vi "Pockels-Initialise sequence for funct acq.vi"(9 "Cluster":T1={"Pockels ON \"Pre\" (samples)"=0, "Direction (+-Inf)"=enum."Toward +Inf", "Additional duration to stay ON (samples)"=0, "Not the last ROI"=FALSE}) -> (1 "Count towards trigger target (ms)":dbl format="%#_9g", 2 "Excess (us)":dbl format="%#_9g", 3 "waveform out":waveform(dbl)(graph))   [LabVIEW 2017]
uses:
  Typedefs/Pockels modulation Internal cluster 1.ctl
  Typedefs/Rounding type.ctl
  Typedefs/Imaging Protocols enum.ctl
  Global Variables/General Globals.vi
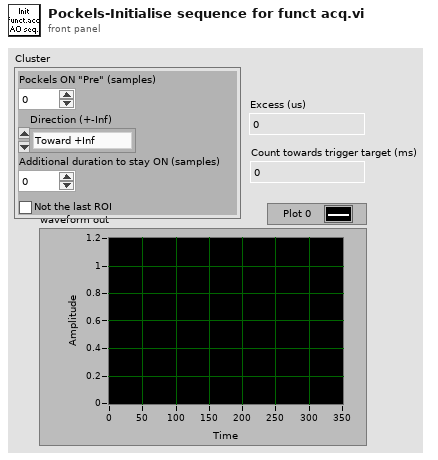
[diagram p1: front panel]
types:
  T1 = typedef "Pockels modulation Internal cluster 1.ctl" = cluster{"Pockels ON \"Pre\" (samples)":i32, "Direction (+-Inf)":T2, "Additional duration to stay ON (samples)":i32, "Not the last ROI":bool}
  T2 = typedef "Rounding type.ctl" = enum16{"No rounding", "Toward +Inf", "Toward -Inf"}
  T3 = typedef "Imaging Protocols enum.ctl" = enum16{"AOL Z-Stack", "Motor Z Stack", "Functional Acquisition", "Single Plane Acquisition", "Volume Acquisition", "Live Imaging", "Live Plane Imaging", "Live Volume Imaging"}
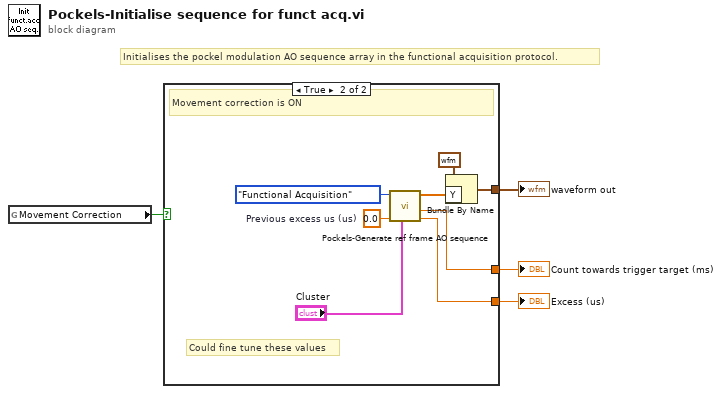
[diagram p0: block diagram]
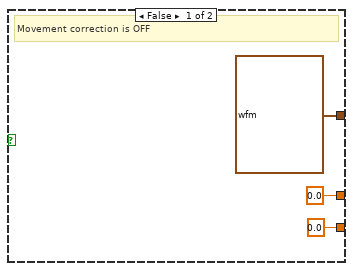
[diagram p2: hidden frame]
diagram:
  # "Initialises the pockel modulation AO sequence array in the functional acquisition protocol."
  n1 = global read "General Globals.vi" "Movement Correction"() -> (w3:bool)
  n2 = case shown="True" w3 {
    tunnel: [waveform(dbl) {"t0"=timestamp(0 s since 1904-01-01), "dt"=0.0, "Y"=[]} ("waveform out") w14] -> w4
    tunnel: [0.0 ("Count towards trigger target (us)") w11] -> w2
    tunnel: [0.0 ("Count towards trigger target (us)") w10] -> w1
    frame False {
      # "Movement correction is OFF"
    }
    frame True {
      w9 = 0.0  # Previous excess us (us)
      # "Could fine tune these values"
      # "Movement correction is ON"
      n3 = call "Pockels-Generate ref frame AO sequence.vi"("Cluster"="Cluster", "Previous excess us (us)"=w9, "Imaging Protocol"=Imaging_Protocols_enum."Functional Acquisition") -> ("Excess (us)"=w10:dbl, "Output sequence length (ms) (corrected for input excess)"=w11:dbl, "Pockels modulation sequence"=w15:dbl[])  [unwired: 4 in, 2 out]
      n4 = Bundle By Name ("Build Waveform")(cluster=waveform(dbl) {"t0"=timestamp(0 s since 1904-01-01), "dt"=0.0, "Y"=[]} ("waveform out"), "Y"=w15) -> (w14:waveform(dbl))
    }
  }
  "waveform out" <- w4
  "Excess (us)" <- w1
  "Count towards trigger target (ms)" <- w2
